vi "FPGA_Index_Rollover_Test.vi"() -> ()   [LabVIEW 2018]
uses:
  <instrlib>/_niInstr/Basic Elements/v1/FPGA/Private/Count Up U32.vi
  <instrlib>/_niInstr/Basic Elements/v1/FPGA/niInstr Basic Elements v1 FPGA.lvlib
panel:
  out "Waveform Chart":cluster{"count out":u32, i32}(graph)
  out "LoopCount":i32
  out "count out":u32
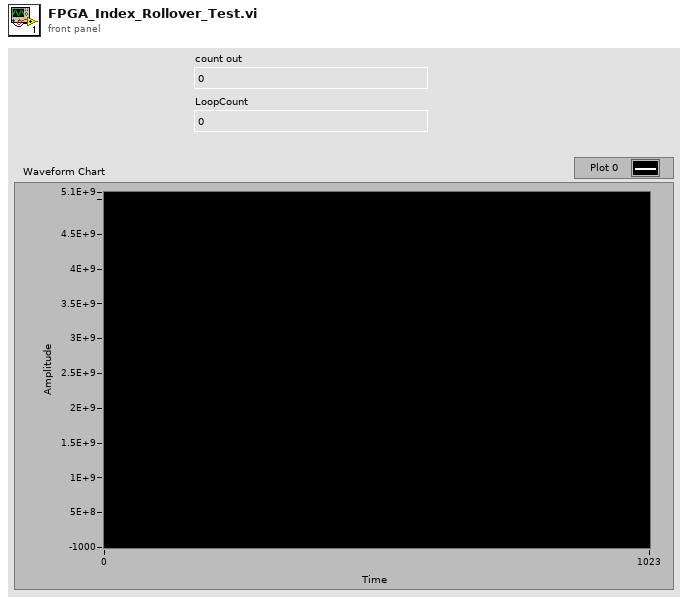
[diagram p1: front panel]
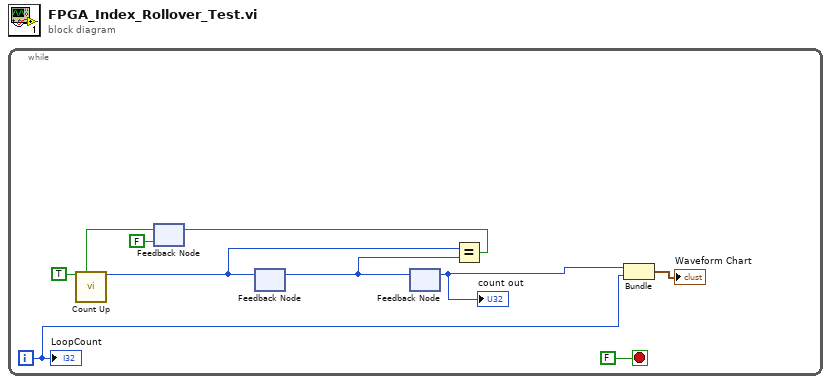
[diagram p0: block diagram]
diagram:
  n1 = while {
    i -> [w4]
    stop <- FALSE stop-if-true
    n2 = feedback #1(FALSE) -> (w8:bool)
    n3 = call-poly <instrlib>:"Count Up.vi"("increment"=TRUE, "reset"=w8) -> ("count out"=w2:u32)  [unwired: 13 in]
    n4 = feedback #2() -> (w1:u32)  [unwired: 1 in]
    n5 = feedback-in #2(w2) -> ()
    n6 = feedback #3() -> (w5:u32)  [unwired: 1 in]
    "count out" <- w5
    n7 = feedback-in #3(w1) -> ()
    n8 = Equal?(x=w2, y=w1) -> (x = y?=w9:bool)
    n9 = feedback-in #1(w9) -> ()
    n10 = Bundle("count out"=w5, w4) -> (→"Waveform Chart":cluster{"count out":u32, i32})  [unwired: 1 in]
    "LoopCount" <- w4
  }
